vi "MTMount_putSample_DeployablePlatforms.vi"(8 "error in (no error)":errorcluster, 11 "Deployable_Platforms_Ctl":T1) -> (0 "error out":errorcluster, 2 "function return":i32, 3 "Deployable_Platforms_Ctl out":T1)   [LabVIEW 2018, in "SALLV_MTMount.lvlib"]
doc: "int MTMount_shm_putSample_Deployable_PlatformsLV(MTMount_Deployable_PlatformsLV *Deployable_Platforms_Ctl );"
uses:
  SALLV_MTMount.lvlib
  DataTypes/Deployable_Platforms.ctl
  SALLV_MTMount.so
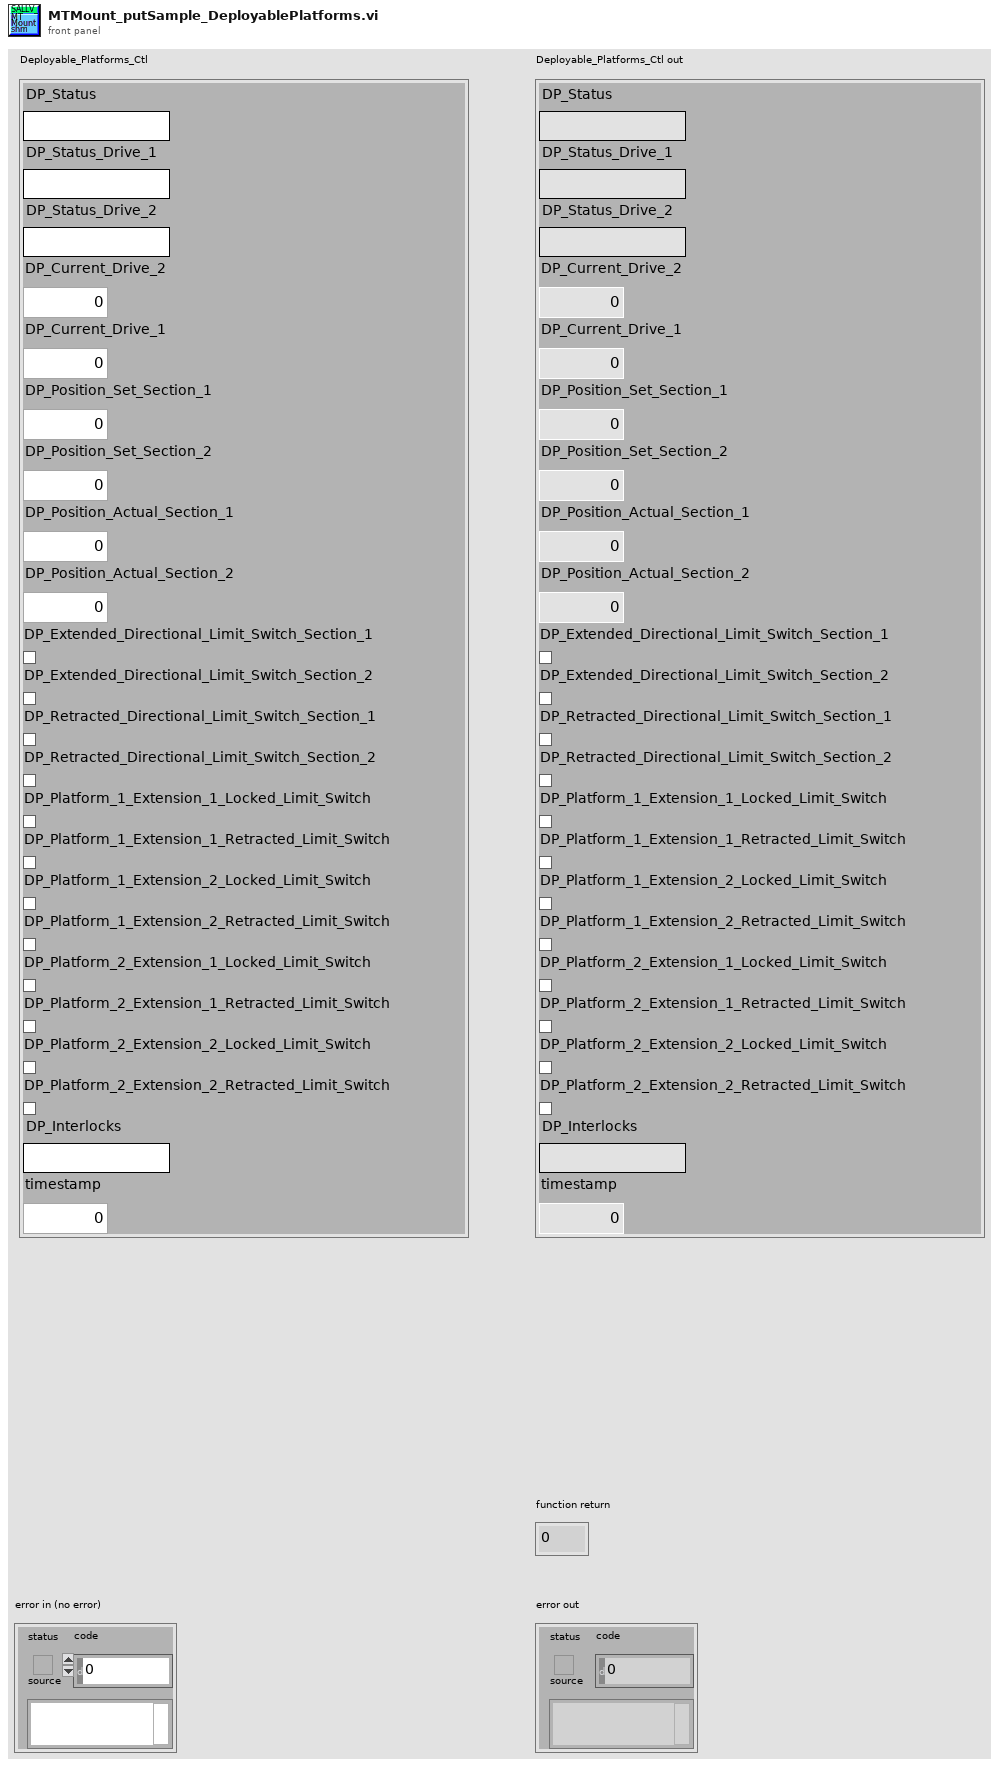
[diagram p1: front panel]
types:
  T1 = typedef "SALLV_MTMount.lvlib/Deployable_Platforms.ctl" = cluster{"DP_Status":string, "DP_Status_Drive_1":string, "DP_Status_Drive_2":string, "DP_Current_Drive_2":dbl, "DP_Current_Drive_1":dbl, "DP_Position_Set_Section_1":dbl, "DP_Position_Set_Section_2":dbl, "DP_Position_Actual_Section_1":dbl, "DP_Position_Actual_Section_2":dbl, "DP_Extended_Directional_Limit_Switch_Section_1":bool, "DP_Extended_Directional_Limit_Switch_Section_2":bool, "DP_Retracted_Directional_Limit_Switch_Section_1":bool, "DP_Retracted_Directional_Limit_Switch_Section_2":bool, "DP_Platform_1_Extension_1_Locked_Limit_Switch":bool, "DP_Platform_1_Extension_1_Retracted_Limit_Switch":bool, "DP_Platform_1_Extension_2_Locked_Limit_Switch":bool, "DP_Platform_1_Extension_2_Retracted_Limit_Switch":bool, "DP_Platform_2_Extension_1_Locked_Limit_Switch":bool, "DP_Platform_2_Extension_1_Retracted_Limit_Switch":bool, "DP_Platform_2_Extension_2_Locked_Limit_Switch":bool, "DP_Platform_2_Extension_2_Retracted_Limit_Switch":bool, "DP_Interlocks":string, "timestamp":dbl}
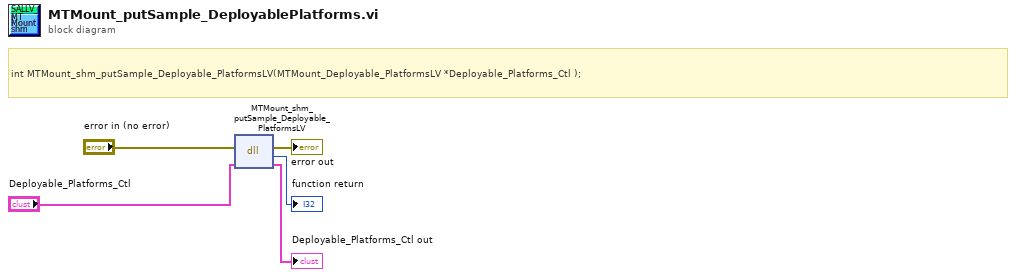
[diagram p0: block diagram]
diagram:
  # "int MTMount_shm_putSample_Deployable_PlatformsLV(MTMount_Deployable_PlatformsLV *Deployable_Platforms_Ctl );"
  n1 = dll-call lib="home/ttsai/Document/salApiMTMount/SALLV_MTMount/SALLV_MTMount.*" fn="MTMount_shm_putSample_Deployable_PlatformsLV"(error in="error in (no error)", "Deployable_Platforms_Ctl"="Deployable_Platforms_Ctl") -> (error out=→"error out":errorcluster, →"function return":i32, "Deployable_Platforms_Ctl"=→"Deployable_Platforms_Ctl out":T1)  [unwired: 2 in, 1 out]
